vi "Riffle Array (CDB).vi"(10 "seed":i32=-1, 11 "X":cdb[](array[numeric])) -> (0 "error":i32, 2 "Riffled Index":i32[](array[numeric]), 3 "Riffled {X}":cdb[](array[numeric]))   [LabVIEW 2018, in "NI_AALBase.lvlib"]
doc: "Riffles the elements in the input array <B>X</B>. Wire data to the <B>X</B> input to determine the polymorphic instance to use or manually select the instance."
uses:
  <vilib>/Analysis/NI_AALBase.lvlib
  <resource>/lvanlys.dll
panel:
  # "Riffle Array (CDB)"
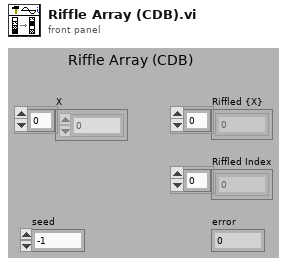
[diagram p1: front panel]
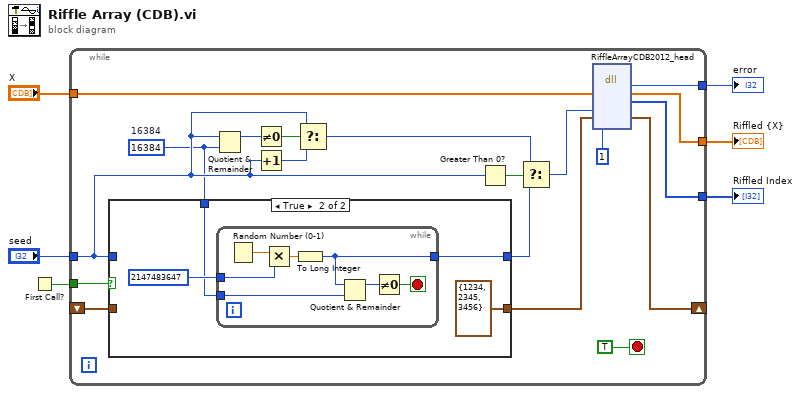
[diagram p0: block diagram]
diagram:
  n1 = First Call?() -> (First Call?: T/F=w6:bool)
  n2 = while {
    tunnel: "seed" -> [w10]
    shift-right: [w18] -> _
    shift-left: _ -> [w23]
    tunnel: w6 -> [w24]
    tunnel: [w22] -> w3
    tunnel: [w21] -> w5
    tunnel: "X" -> [w20]
    tunnel: [w17] -> w1
    stop <- TRUE stop-if-true
    w7 = 16384  # 16384
    n3 = case shown="True" w24 {
      tunnel: w23 -> [w27 _]
      tunnel: [w27 cluster{"xSeed":i32, "ySeed":i32, "zSeed":i32} {"xSeed"=1234, "ySeed"=2345, "zSeed"=3456} ("RNGState")] -> w19
      tunnel: [w26 w28] -> w9
      tunnel: w10 -> [w26 _]
      tunnel: w7 -> [_ w29]
      frame False {
      }
      frame True {
        n4 = while {
          tunnel: [w36] -> w28
          tunnel: w29 -> [w35]
          tunnel: 2147483647 ("x") -> [w32]
          stop <- w33 stop-if-true
          n5 = Random Number (0-1)() -> (number: 0 to 1=w37:dbl)
          n6 = Multiply(x=w37, y=w32) -> (x*y=w38:dbl)
          n7 = To Long Integer(number=w38) -> (32bit integer=w36:i32)
          n8 = Quotient & Remainder(x=w36, y=w35) -> (x-y*floor(x/y)=w34:i32)  [unwired: 1 out]
          n9 = Not Equal To 0?(x=w34) -> (x != 0?=w33:bool)
        }
      }
    }
    n10 = Quotient & Remainder(x=w10, y=w7) -> (x-y*floor(x/y)=w14:i32)  [unwired: 1 out]
    n11 = Not Equal To 0?(x=w14) -> (x != 0?=w13:bool)
    n12 = Increment(x=w10) -> (x+1=w12:i32)
    n13 = Select(t=w10, s=w13, f=w12) -> (s? t:f=w11:i32)
    n14 = Greater Than 0?(x=w10) -> (x > 0?=w15:bool)
    n15 = Select(t=w11, s=w15, f=w9) -> (s? t:f=w8:i32)
    n16 = dll-call lib="C:/Program Files (x86)/National Instruments/LabVIEW 2018/resource/lvanlys.*" fn="RiffleArrayCDB2012_head"("riffle"=w20, "seed"=w8, "rngState"=w19, "option"=1) -> ("return type"=w22:i32, "riffle"=w21:cdb[], "riffleIndex"=w17:i32[], "rngState"=w18:cluster{"xSeed":i32, "ySeed":i32, "zSeed":i32})  [unwired: 6 in, 2 out]
  }
  "Riffled {X}" <- w5
  "error" <- w3
  "Riffled Index" <- w1
